vi "S2DS_Choose Scipt File.vi"() -> ()   [LabVIEW 2025]
uses:
  <vilib>/Utility/sysdir.llb/System Directory Type.ctl
  <vilib>/Utility/config.llb/Read Key (Path).vi
  <vilib>/Utility/config.llb/Write Key (Path).vi
  <vilib>/Utility/config.llb/Write Key (I32).vi
  <vilib>/Utility/config.llb/NI_LVConfig.lvlib
panel:
  in  "stop":bool
  in  "Select the script file...":path
  # "Select the script file..."
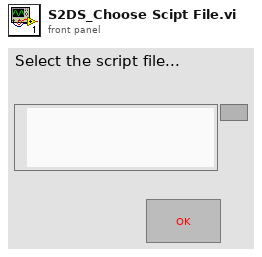
[diagram p1: front panel]
types:
  T1 = typedef "System Directory Type.ctl" = i32
  T2 = typedef "NI_LVConfig.lvlib/Config Data RefNum.ctl" = refnum<k1>
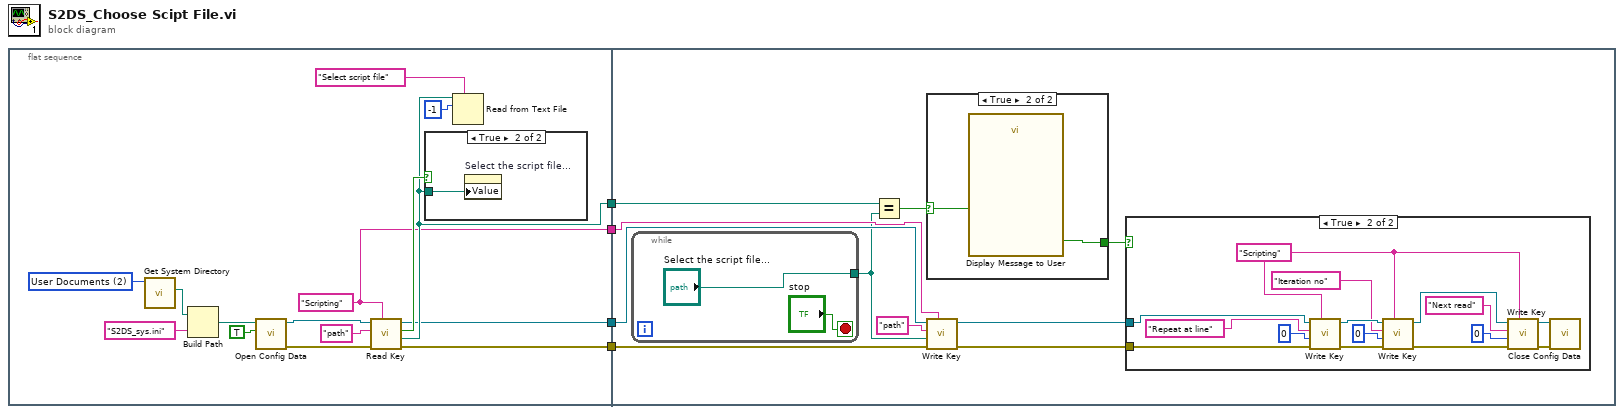
[diagram p0: block diagram]
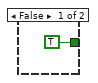
[diagram p4: hidden frame]
diagram:
  n1 = flat-sequence {
    tunnel: [w8] -> w4
    tunnel: [w7] -> w3
    tunnel: [w6] -> w2
    tunnel: [w5] -> w1
    tunnel: w4 -> [w30]
    tunnel: w3 -> [w27]
    tunnel: w2 -> [w25]
    tunnel: w1 -> [w23]
    frame #0 {
      w5 = "Scripting" ("section")
      w16 = T1 2 items=["User Home"=0, "User Desktop"=1, "User Documents"=2, "User Application Data"=3, "User Preferences"=4, "User Temporary"=5, "Public Documents"=6, "Public Application Data"=7, "Public Preferences"=8, "Public Cache"=13, "System Core Libraries"=9, "System Installed Libraries"=10, "Application Files"=11, "Boot Volume Root"=12] ("system directory type")
      n2 = call <vilib>:"Get System Directory.vi"("system directory type"=w16) -> ("system directory"=w15:path)  [unwired: 10 in]
      n3 = Build Path(base path=w15, name or relative path="S2DS_sys.ini") -> (appended path=w13:path)
      n4 = call <vilib>:"Open Config Data.vi"("create file if necessary (T)"=TRUE, "configuration file path"=w13) -> ("error out"=w11:errorcluster, "refnum"=w12:T2)  [unwired: 7 in, 1 out]
      n5 = call-poly <vilib>:"Read Key.vi"("section"=w5, "error in (no error)"=w11, "key"="path", "refnum"=w12) -> ("error out"=w6:errorcluster, "value"=w8:path, "found?"=w9:bool, "refnum out"=w7:T2)  [unwired: 4 in]
      n6 = case shown="True" w9 {
        tunnel: w8 -> [_ w20]
        frame False {
        }
        frame True {
          n7 = property on="Select the script file..." class="Path"("Value"=w20) -> ()  [unwired: 2 in, 2 out]
        }
      }
      n8 = Read from Text File(prompt (Open existing file)="Select script file" ("prompt"), file (use dialog)=w8, count=-1) -> ()  [unwired: 1 in, 4 out]
    }
    frame #1 {
      n9 = while {
        tunnel: ["Select the script file..."] -> w21
        stop <- "stop" stop-if-true
      }
      n10 = Equal?(x=w30, y=w21) -> (x = y?=w29:bool)
      n11 = case shown="True" w29 {
        selector: w29 -> [_ w48]
        tunnel: [TRUE w47] -> w28
        frame False {
        }
        frame True {
          n12 = call "Display Message to User"("Enable"=w48) -> ("YES, start over."=w47:bool)  [unwired: 9 in, 1 out]
        }
      }
      n13 = call-poly <vilib>:"Write Key.vi"("section"=w23, "error in (no error)"=w25, "value"=w21, "key"="path", "refnum"=w27) -> ("error out"=w24:errorcluster, "refnum out"=w26:T2)  [unwired: 4 in, 1 out]
      n14 = case shown="True" w28 {
        tunnel: w26 -> [_ w35]
        tunnel: w24 -> [_ w34]
        frame False {
        }
        frame True {
          w39 = "Scripting" ("section")
          n15 = call-poly <vilib>:"Write Key.vi"("section"=w39, "error in (no error)"=w34, "value"=0, "key"="Repeat at line", "refnum"=w35) -> ("error out"=w43:errorcluster, "refnum out"=w44:T2)  [unwired: 4 in, 1 out]
          n16 = call-poly <vilib>:"Write Key.vi"("section"=w39, "error in (no error)"=w43, "value"=0, "key"="Iteration no", "refnum"=w44) -> ("error out"=w40:errorcluster, "refnum out"=w41:T2)  [unwired: 4 in, 1 out]
          n17 = call-poly <vilib>:"Write Key.vi"("section"=w39, "error in (no error)"=w40, "value"=0, "key"="Next read", "refnum"=w41) -> ("error out"=w36:errorcluster, "refnum out"=w37:T2)  [unwired: 4 in, 1 out]
          n18 = call <vilib>:"Close Config Data.vi"("error in (no error)"=w36, "refnum"=w37) -> ()  [unwired: 8 in, 2 out]
        }
      }
    }
  }
